vi "Run_TestFailure_CallsListenerAddFailure.vi"() -> ()   [LabVIEW 2019, in "TestResultTest.lvlib"]
uses:
  TestResultTest.lvlib
  TestResult/TestResult.lvclass
  Support/TestCaseMock/TestCaseMock.lvclass/TestCaseMock.ctl
  Support/FakeTestListener/FakeTestListener.lvclass
  C:/Users/de200256/Code/LVUnit/TestListener/TestListener.lvclass
  Support/TestCaseMock/TestCaseMock.lvclass
  C:/Users/de200256/Code/LVUnit/TestCase/TestCase/TestCase.lvclass
  Assertion/Assertion.lvlib
  C:/Users/de200256/Code/LVUnit/Test/Test.lvclass
panel:
  out "error out":errorcluster
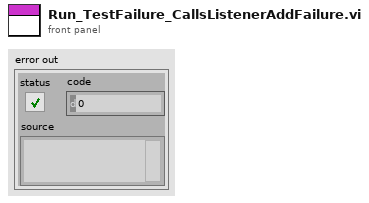
[diagram p1: front panel]
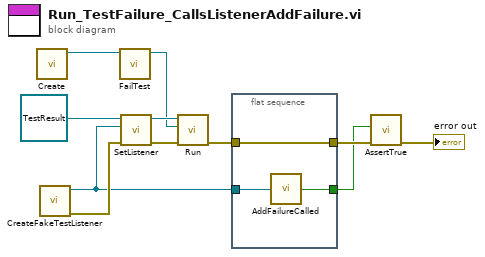
[diagram p0: block diagram]
diagram:
  n1 = call "Create.vi"() -> ("TestCaseMock"=w2:refnum<class "TestCaseMock.lvclass">)  [unwired: 10 in, 1 out]
  n2 = call "CreateFakeTestListener.vi"() -> ("error out"=w10:errorcluster, "FakeTestListener"=w9:refnum<class "FakeTestListener.lvclass">)  [unwired: 10 in]
  n3 = call "FailTest.vi"("TestCaseMock in"=w2) -> ("TestCaseMock out"=w1:refnum<class "TestCaseMock.lvclass">)  [unwired: 10 in]
  n4 = call "SetListener.vi"("error in (no error)"=w10, "Listener"=w9, "TestResult in"=refnum<class "TestResult.lvclass"> refnum ("TestResult.lvclass")) -> ("error out"=w8:errorcluster, "TestResult in"=w6:refnum<class "TestResult.lvclass">)  [unwired: 7 in]
  n5 = call-dynamic "Run.vi"("error in (no error)"=w8, "TestCase"=w1, "TestResult in"=w6) -> ("error out"=w7:errorcluster)  [unwired: 6 in, 2 out]
  n6 = flat-sequence {
    tunnel: w9 -> [w14]
    tunnel: w7 -> [w13]
    tunnel: [w13] -> w4
    tunnel: [w12] -> w3
    frame #0 {
      n7 = call "AddFailureCalled.vi"("FakeTestListener In"=w14) -> ("AddFailure Called"=w12:bool)
    }
  }
  n8 = call "AssertTrue.vi"("error in (no error)"=w4, "Condition"=w3) -> ("error out"=→"error out":errorcluster)  [unwired: 9 in]
